vi "Update Node Shape.vi"(0 "Edges":refnum<class "FSM.Edge.lvclass">[](array[class]), 7 "FSM.Node in":refnum<class "FSM.Node.lvclass">) -> (4 "Edges Out":refnum<class "FSM.Edge.lvclass">[](array[class]), 8 "FSM.Node out":refnum<class "FSM.Node.lvclass">)   [LabVIEW 2020, in "FSM.Graph.lvclass"]
uses:
  FSM.Graph.lvclass
  FSM.Node/FSM.Node.lvclass
  FSM.Edge/FSM.Edge.lvclass
  FSM.Node/FSM.Node.lvclass/FSM.Node.ctl
  FSM.Edge/FSM.Edge.lvclass/FSM.Edge.ctl
  FSM.Node/Shape.ctl
  FSM.Edge/Read SourceName.vi
  FSM.Node/Write Shape.vi
  FSM.Node/Read Shape.vi
  FSM.Node/Read Name.vi
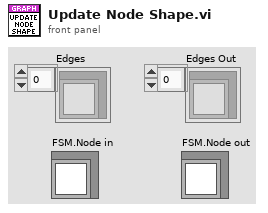
[diagram p1: front panel]
types:
  T1 = typedef "FSM.Node.lvclass/Shape.ctl" = enum16{"Default", "Start", "Action", "End"}
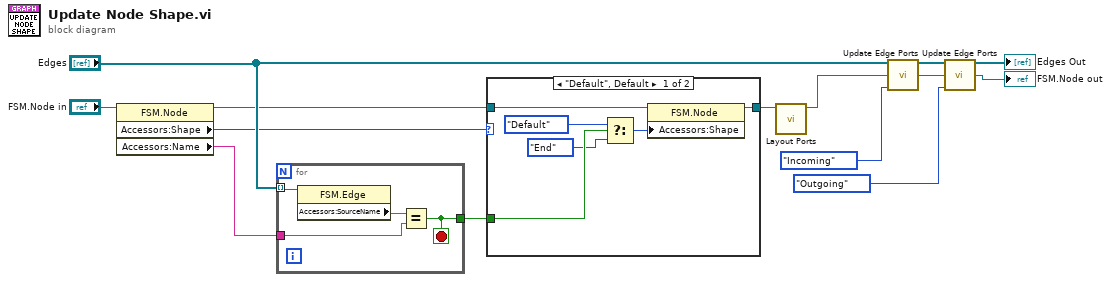
[diagram p0: block diagram]
diagram:
  n1 = property class="FSM.Node"(reference="FSM.Node in") -> (reference out=w8:refnum<class "FSM.Node.lvclass">, "Accessors:Shape"=w1:T1, "Accessors:Name"=w2:string)  [unwired: 1 in, 1 out]
  n2 = for {
    tunnel: "Edges" -> [w18] mode=indexing
    tunnel: w2 -> [w16]
    tunnel: [w15] -> w12
    stop <- w15 stop-if-true
    n3 = property class="FSM.Edge"(reference=w18) -> ("Accessors:SourceName"=w17:string)  [unwired: 1 in, 2 out]
    n4 = Equal?(x=w17, y=w16) -> (x = y?=w15:bool)
  }
  n5 = case shown="\"Default\", Default" w1 {
    tunnel: w12 -> [w24 _]
    tunnel: [w23 w25] -> w10
    tunnel: w8 -> [w19 w25]
    frame "Default", Default {
      n6 = Select(t=Shape."Default" ("Shape"), s=w24, f=Shape."End") -> (s? t:f=w22:T1)
      n7 = property class="FSM.Node"(reference=w19, "Accessors:Shape"=w22) -> (reference out=w23:refnum<class "FSM.Node.lvclass">)  [unwired: 1 in, 1 out]
    }
    frame "Start" {
    }
  }
  n8 = call "Layout Ports.vi"("Node in"=w10) -> ("Node out"=w13:refnum<class "FSM.Node.lvclass">)  [unwired: 9 in, 1 out]
  n9 = call "Update Edge Ports.vi"("Edges In"="Edges", "FSM.Node In"=w13, "Edges"=enum16{"Incoming", "Outgoing"}."Incoming") -> ("Edges Out"=w7:refnum<class "FSM.Edge.lvclass">[], "FSM.Node thru"=w6:refnum<class "FSM.Node.lvclass">)  [unwired: 11 in]
  n10 = call "Update Edge Ports.vi"("Edges In"=w7, "FSM.Node In"=w6, "Edges"=enum16{"Incoming", "Outgoing"}."Outgoing") -> ("Edges Out"=→"Edges Out":refnum<class "FSM.Edge.lvclass">[], "FSM.Node thru"=→"FSM.Node out":refnum<class "FSM.Node.lvclass">)  [unwired: 11 in]
